vi "Set Current Range.vi"(0 "VISA resource name":refnum<visa-resource-name>="GPIB0::24::INSTR", 5 "Range":dbl, 11 "error in (no error)":errorcluster) -> (4 "VISA resource name out":refnum<visa-resource-name>="GPIB0::24::INSTR", 15 "error out":errorcluster)   [LabVIEW 2010]
uses:
  <instrlib>/Keithley 24XX/Keithley 24XX.lvlib
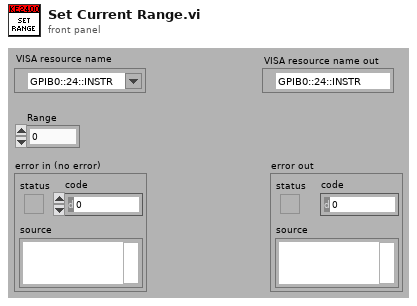
[diagram p1: front panel]
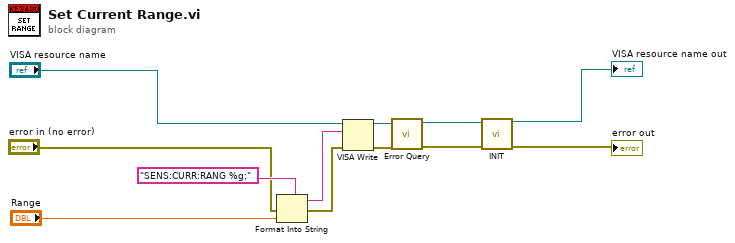
[diagram p0: block diagram]
diagram:
  n1 = Format Into String(format string="SENS:CURR:RANG %g;" ("Manual Range"), error in="error in (no error)", "Range") -> (resulting string=w5:string, error out=w4:errorcluster)  [unwired: 1 in]
  n2 = VISA Write(VISA resource name="VISA resource name", write buffer=w5, error in (no error)=w4) -> (VISA resource name out=w9:refnum<visa-resource-name>, error out=w8:errorcluster)  [unwired: 1 out]
  n3 = call <instrlib>:"Error Query.vi"("error in (no error)"=w8, "VISA resource name"=w9) -> ("error out"=w10:errorcluster, "VISA resource name out"=w7:refnum<visa-resource-name>)  [unwired: 6 in, 2 out]
  n4 = call "INIT.vi"("VISA resource name"=w7, "error in (no error)"=w10) -> ("VISA resource name out"=→"VISA resource name out":refnum<visa-resource-name>, "error out"=→"error out":errorcluster)  [unwired: 12 in]
